vi "JSONtext Help.vi"   [LabVIEW 2019]
uses:
  <vilib>/Platform/browser.llb/Open URL in Default Browser (path).vi
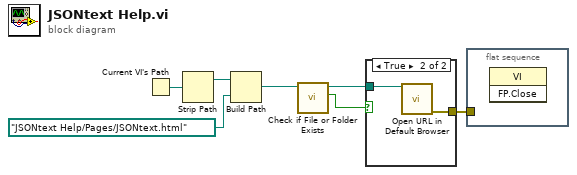
[diagram p0: block diagram]
diagram:
  n1 = Current VI's Path() -> (path=w6:path)
  n2 = Strip Path(path=w6) -> (stripped path=w5:path)  [unwired: 1 out]
  n3 = Build Path(base path=w5, name or relative path=path "JSONtext Help/Pages/JSONtext.html" ("path")) -> (appended path=w3:path)
  n4 = call <vilib>:"Check if File or Folder Exists.vi"("path"=w3) -> ("file or folder exists?"=w1:bool, "dup path"=w2:path)  [unwired: 8 in, 1 out]
  n5 = case shown="True" w1 {
    tunnel: [_ w9] -> w4
    tunnel: w2 -> [_ w8]
    frame False {
    }
    frame True {
      n6 = call-poly <vilib>:"Open URL in Default Browser.vi"("path"=w8) -> ("error out"=w9:errorcluster)  [unwired: 5 in, 1 out]
    }
  }
  n7 = flat-sequence {
    tunnel: w4 -> [_]
    frame #0 {
      n8 = invoke class="VI" method="FP.Close"() -> ()  [unwired: 3 in, 3 out]
    }
  }
